vi "Create All Message Queues.vi"(8 "error in (no error)":errorcluster) -> (0 "error out":errorcluster, 3 "Message Queues out":T1)   [LabVIEW 2017, in "Message Queue.lvlib"]
doc: "This VI creates and initializes all the message queues for your application. If your application requires more than one message queue, right-click the \"Message Queues\" constant above and select Open Type Def. Add the new Message Queue(s) to the type definition, then initialize them in this VI."
uses:
  Message Queue.lvlib
  All Message Queues.ctl
  Message Cluster.ctl
  Enqueue Message (Single).vi
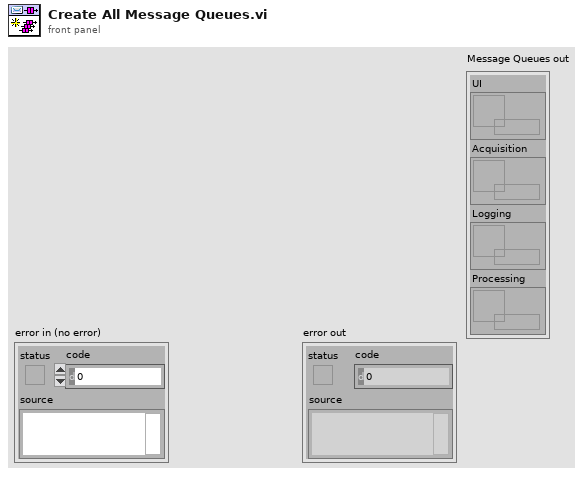
[diagram p1: front panel]
types:
  T1 = typedef "Message Queue.lvlib/All Message Queues.ctl" = cluster{"UI":refnum<queue>, "Acquisition":refnum<queue>, "Logging":refnum<queue>, "Processing":refnum<queue>}
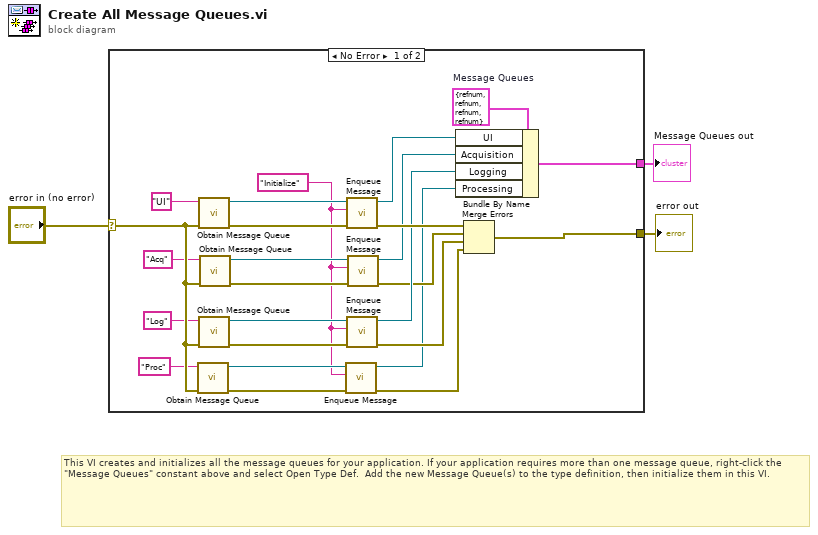
[diagram p0: block diagram]
diagram:
  # "This VI creates and initializes all the message queues for your application. If your application requires more than one message queue, right-click the \"Message Queues\" constant above and select Open Type Def.  Add the new Message Queue(s) to the type definition, then initialize them in this VI."
  n1 = case shown="No Error" "error in (no error)" {
    selector: "error in (no error)" -> [w11 w29]
    tunnel: [w16 w29] -> w3
    tunnel: [w26 _] -> w2
    frame No Error {
      w8 = "Initialize" ("Message")
      w27 = T1 {"UI"=refnum, "Acquisition"=refnum, "Logging"=refnum, "Processing"=refnum}  # Message Queues
      n2 = call "Obtain Message Queue.vi"("error in (no error)"=w11, "name (unnamed)"="Proc") -> ("error out"=w12:errorcluster, "Message Queue"=w13:refnum<queue>)  [unwired: 8 in]
      n3 = call "Obtain Message Queue.vi"("error in (no error)"=w11, "name (unnamed)"="UI") -> ("error out"=w25:errorcluster, "Message Queue"=w24:refnum<queue>)  [unwired: 8 in]
      n4 = call "Obtain Message Queue.vi"("error in (no error)"=w11, "name (unnamed)"="Log") -> ("error out"=w21:errorcluster, "Message Queue"=w20:refnum<queue>)  [unwired: 8 in]
      n5 = call "Obtain Message Queue.vi"("error in (no error)"=w11, "name (unnamed)"="Acq") -> ("error out"=w22:errorcluster, "Message Queue"=w23:refnum<queue>)  [unwired: 8 in]
      n6 = call-poly "Enqueue Message.vi"("error in (no error)"=w12, "Message"=w8, "Message Queue"=w13) -> ("error out"=w10:errorcluster, "dup Message Queue"=w9:refnum<queue>)  [unwired: 7 in]
      n7 = call-poly "Enqueue Message.vi"("error in (no error)"=w25, "Message"=w8, "Message Queue"=w24) -> ("error out"=w28:errorcluster, "dup Message Queue"=w19:refnum<queue>)  [unwired: 7 in]
      n8 = call-poly "Enqueue Message.vi"("error in (no error)"=w21, "Message"=w8, "Message Queue"=w20) -> ("error out"=w14:errorcluster, "dup Message Queue"=w17:refnum<queue>)  [unwired: 7 in]
      n9 = call-poly "Enqueue Message.vi"("error in (no error)"=w22, "Message"=w8, "Message Queue"=w23) -> ("error out"=w15:errorcluster, "dup Message Queue"=w18:refnum<queue>)  [unwired: 7 in]
      n10 = Bundle By Name(cluster=w27, "UI"=w19, "Acquisition"=w18, "Logging"=w17, "Processing"=w9) -> (w26:T1)
      n11 = Merge Errors(w28, w15, w14, w10) -> (w16:errorcluster)
    }
    frame Error {
    }
  }
  "Message Queues out" <- w2
  "error out" <- w3
